vi "GenerateData.vi"(8 "error in (no error)":errorcluster, 11 "DemoDAQ in":refnum<class "DemoDAQ.lvclass">) -> (0 "error out":errorcluster, 2 "DataExchange":T2, 3 "DemoDAQ out":refnum<class "DemoDAQ.lvclass">)   [LabVIEW 2020, in "DemoDAQ.lvlib" / "DemoDAQ.lvclass"]
uses:
  DemoDAQ.lvclass
  Hardware Abstraction Layer/Component/Device/Device/DataExchange.ctl
  DemoDAQ.lvclass/DemoDAQ.ctl
  Hardware Abstraction Layer/Component/DAQ/DAQ/DAQ.lvclass
  Interface/DataListener/DataListener.lvclass
panel:
  in  "Cluster":T1 {"QPD  Sum" format="%#_13g"; "QPD Voltage Y" format="%#_13g"; "QPD Voltage X" format="%#_13g"}
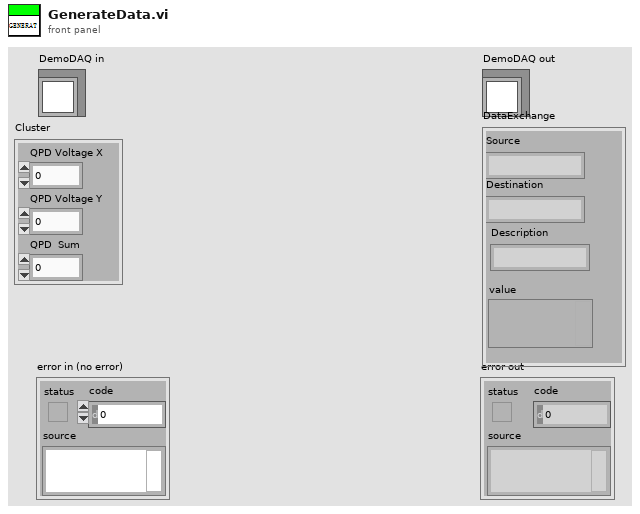
[diagram p1: front panel]
types:
  T1 = cluster{"QPD Voltage X":dbl, "QPD Voltage Y":dbl, "QPD  Sum":dbl}
  T2 = typedef "DataListener.lvclass/DataExchange.ctl" = cluster{"Source":string, "Destination":string, "Description":string, "value":variant}
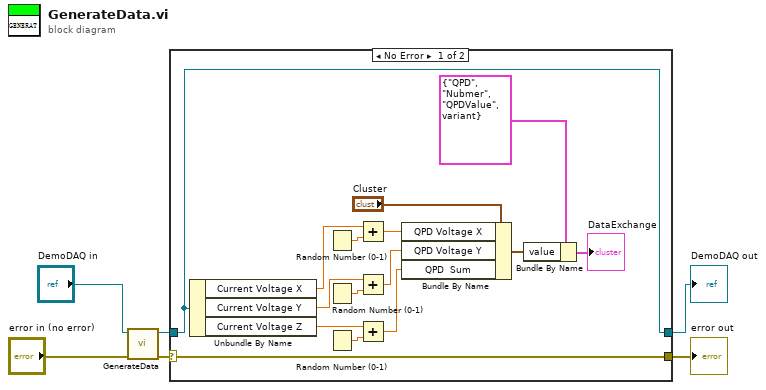
[diagram p0: block diagram]
diagram:
  n1 = call-parent "GenerateData.vi"("error in (no error)"="error in (no error)", "Device in"="DemoDAQ in") -> ("error out"=w4:errorcluster, "Device out"=w2:refnum<class "DemoDAQ.lvclass">)  [unwired: 7 in, 1 out]
  n2 = case shown="No Error" w4 {
    selector: w4 -> [w21 w23]
    tunnel: [w21 w23] -> w3
    tunnel: w2 -> [w20 w22]
    tunnel: [w20 w22] -> w1
    frame No Error {
      n3 = Unbundle By Name(w20) -> ("Current Voltage X"=w19:dbl, "Current Voltage Y"=w17:dbl, "Current Voltage Z"=w15:dbl)
      n4 = Random Number (0-1)() -> (number: 0 to 1=w18:dbl)
      n5 = Random Number (0-1)() -> (number: 0 to 1=w16:dbl)
      n6 = Random Number (0-1)() -> (number: 0 to 1=w14:dbl)
      n7 = Add(x=w19, y=w18) -> (x+y=w9:dbl)
      n8 = Add(x=w17, y=w16) -> (x+y=w8:dbl)
      n9 = Add(x=w15, y=w14) -> (x+y=w7:dbl)
      n10 = Bundle By Name(cluster="Cluster", "QPD Voltage X"=w9, "QPD Voltage Y"=w8, "QPD  Sum"=w7) -> (w10:T1)
      n11 = Bundle By Name(cluster=T2 {"Source"="QPD", "Destination"="Nubmer", "Description"="QPDValue", "value"=variant} ("DataExchange"), "value"=w10) -> (→"DataExchange":T2)
    }
    frame Error {
    }
  }
  "error out" <- w3
  "DemoDAQ out" <- w1
